vi "CMI Sync V3 Get Channel Timestamp.vi"(8 "error in":errorcluster, 10 "Channel (1)":i32=1 min=1 max=2 step=1, 11 "session in":T1={"VISA"="", "baud rate [bd/s]"=115200, "source"=enum."Auto", "hv range"=enum."1kV", "fsrc is fixed"=FALSE, "fsrc [Hz]"=10000000.0, "freq integ [s]"=1.0, "freq filter"=5, "trig level"=enum."TTL 5V", "chn1 mode"=enum."Source divider", "chn1 level"=enum."Positive 5V", "chn2 mode"=enum."Source divider", "chn2 level"=enum."Positive 5V", "chn2 div"=1, "chn3 mode"=enum."Chn 1 Active", "chn3 level"=enum."Positive 5V"} {"chn2 div" min=1 max=100000000 step=1; "fsrc [Hz]" format="%_8p"}) -> (0 "error out":errorcluster, 2 "timestamp [s]":dbl, 3 "session out":T1={"VISA"="", "baud rate [bd/s]"=115200, "source"=enum."Auto", "hv range"=enum."1kV", "fsrc is fixed"=FALSE, "fsrc [Hz]"=10000000.0, "freq integ [s]"=1.0, "freq filter"=5, "trig level"=enum."TTL 5V", "chn1 mode"=enum."Source divider", "chn1 level"=enum."Positive 5V", "chn2 mode"=enum."Source divider", "chn2 level"=enum."Positive 5V", "chn2 div"=1, "chn3 mode"=enum."Chn 1 Active", "chn3 level"=enum."Positive 5V"} {"chn2 div" min=1 max=100000000 step=1; "fsrc [Hz]" format="%_8p"})   [LabVIEW 2020, in "AWG.lvlib" / "CMI Sync Unit V3.lvlib"]
doc: "Reads channel 1 or 2 trigger timestamp."
uses:
  CMI Sync Unit V3.lvlib
  CMI Sync V3 session.ctl
  Configure/CMI Sync V3 Reference Clock Source.ctl
  Configure/CMI Sync V3 HV input Range.ctl
  Configure/CMI Sync V3 Trigger Input Level.ctl
  Configure/CMI Sync V3 Channel 1 Mode.ctl
  Configure/CMI Sync V3 Channel Output Levels.ctl
  Configure/CMI Sync V3 Channel 2 Mode.ctl
  Configure/CMI Sync V3 Channel 3 Mode.ctl
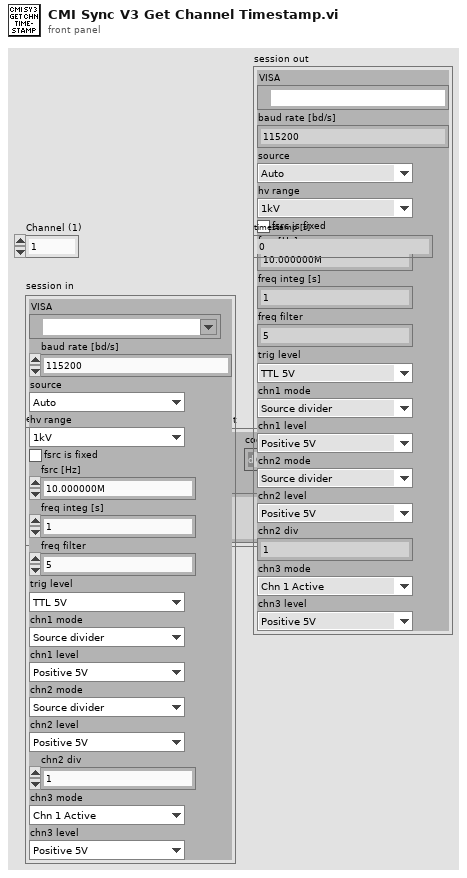
[diagram p1: front panel]
types:
  T1 = typedef "AWG.lvlib/CMI Sync Unit V3.lvlib/CMI Sync V3 session.ctl" = cluster{"VISA":refnum<visa-resource-name>, "baud rate [bd/s]":i32, "source":T2, "hv range":T3, "fsrc is fixed":bool, "fsrc [Hz]":dbl, "freq integ [s]":dbl, "freq filter":i32, "trig level":T4, "chn1 mode":T5, "chn1 level":T6, "chn2 mode":T7, "chn2 level":T6, "chn2 div":i32, "chn3 mode":T8, "chn3 level":T6}
  T2 = typedef "AWG.lvlib/CMI Sync Unit V3.lvlib/CMI Sync V3 Reference Clock Source.ctl" = enum16{"Auto", "Internal", "Logic", "Sine", "HV"}
  T3 = typedef "AWG.lvlib/CMI Sync Unit V3.lvlib/CMI Sync V3 HV input Range.ctl" = enum16{"10V", "60V", "250V", "1kV"}
  T4 = typedef "AWG.lvlib/CMI Sync Unit V3.lvlib/CMI Sync V3 Trigger Input Level.ctl" = enum16{"LVCMOS 3V3", "TTL 5V"}
  T5 = typedef "AWG.lvlib/CMI Sync Unit V3.lvlib/CMI Sync V3 Channel 1 Mode.ctl" = enum16{"Source divider", "DDS absolute", "DDS ratio", "DDS ratio M/N"}
  T6 = typedef "AWG.lvlib/CMI Sync Unit V3.lvlib/CMI Sync V3 Channel Output Levels.ctl" = enum16{"Positive 3V3", "Negative 3V3", "Positive 5V", "Negative 5V"}
  T7 = typedef "AWG.lvlib/CMI Sync Unit V3.lvlib/CMI Sync V3 Channel 2 Mode.ctl" = enum16{"Source divider", "Chn 1 divide"}
  T8 = typedef "AWG.lvlib/CMI Sync Unit V3.lvlib/CMI Sync V3 Channel 3 Mode.ctl" = enum16{"Chn 1 Active", "Chn 2 Active", "Chn 1 Trigger", "Chn 2 Trigger", "Gate", "PPS", "10MHz"}
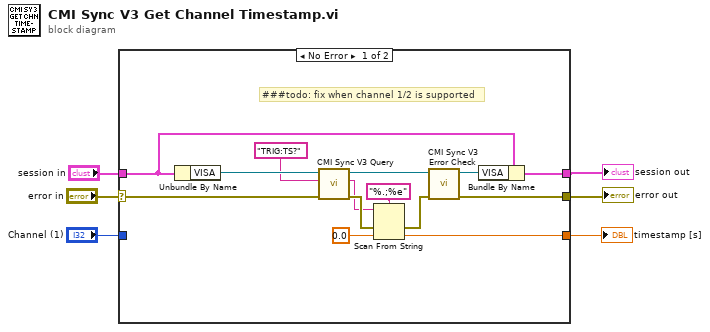
[diagram p0: block diagram]
diagram:
  n1 = case shown="No Error" "error in" {
    selector: "error in" -> [w8 w22]
    tunnel: "session in" -> [w20 w21]
    tunnel: [w19 w21] -> w1
    tunnel: [w17 w22] -> w2
    tunnel: "Channel (1)" -> [_ _]
    tunnel: [w9 _] -> w3
    frame No Error {
      # "###todo: fix when channel 1/2 is supported"
      n2 = Unbundle By Name(w20) -> ("VISA"=w16:refnum<visa-resource-name>)
      n3 = call "CMI Sync V3 Query.vi"("error in"=w8, "command"="TRIG:TS?" ("format string"), "VISA in"=w16) -> ("error out"=w14:errorcluster, "read buffer"=w11:string, "VISA resource name out"=w15:refnum<visa-resource-name>)  [unwired: 6 in]
      n4 = Scan From String(format string="%.;%e", input string=w11, error in=w14, default 1=0.0 ("default value 1")) -> (error out=w13:errorcluster, output 1=w9:dbl)  [unwired: 1 in, 2 out]
      n5 = call "CMI Sync V3 Error Check.vi"("error in"=w13, "VISA in"=w15) -> ("error out"=w17:errorcluster, "VISA out"=w18:refnum<visa-resource-name>)  [unwired: 7 in, 1 out]
      n6 = Bundle By Name(cluster=w20, "VISA"=w18) -> (w19:T1)
    }
    frame Error {
    }
  }
  "error out" <- w2
  "session out" <- w1
  "timestamp [s]" <- w3
